vi "Git_UpdateApplicationPrep.vi"   [LabVIEW 2012]
uses:
  <vilib>/httpClient/LabVIEWHTTPClient.lvlib
  <vilib>/zip/NI_Unzip.lvlib
types:
  T1 = typedef "LabVIEWHTTPClient.lvlib/ClientHandle.ctl" = refnum<k1>
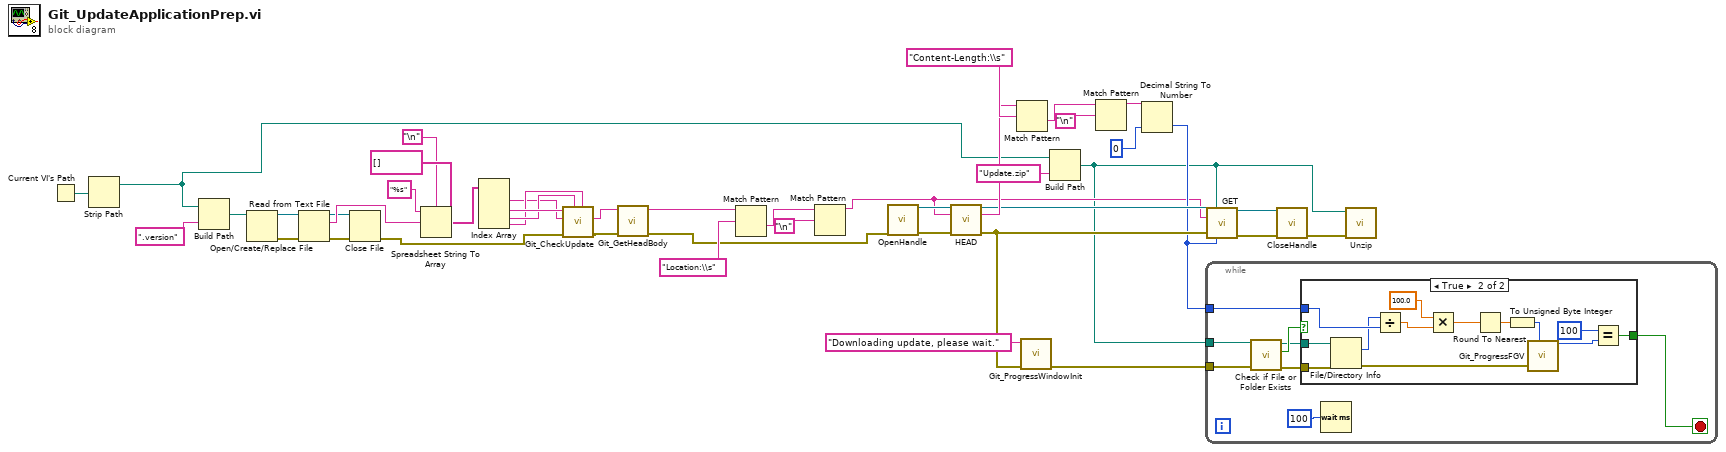
[diagram p0: block diagram]
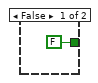
[diagram p2: hidden frame]
diagram:
  n1 = Current VI's Path() -> (path=w37:path)
  n2 = Strip Path(path=w37) -> (stripped path=w1:path)  [unwired: 1 out]
  n3 = Build Path(base path=w1, name or relative path=".version") -> (appended path=w43:path)
  n4 = Open/Create/Replace File(file path (use dialog)=w43) -> (refnum out=w41:refnum<file>, error out=w42:errorcluster)  [unwired: 5 in, 1 out]
  n5 = Read from Text File(file (use dialog)=w41, error in=w42) -> (refnum out=w29:refnum<file>, text=w39:string, error out=w31:errorcluster)  [unwired: 2 in, 1 out]
  n6 = Close File(refnum=w29, error in=w31) -> (error out=w30:errorcluster)  [unwired: 1 out]
  n7 = Spreadsheet String To Array(delimiter (Tab)="\n", format string="%s", spreadsheet string=w39, array type (2D Dbl)=string[] []) -> (array=w35:string[])
  n8 = Index Array(array=w35) -> (element #1=w28:string, element #2=w34:string, element #3=w33:string, element #4=w32:string)  [unwired: 4 in]
  n9 = call "Git_CheckUpdate.vi"("Current Version Date (YYYY-MM-DD)"=w32, "Current Version Number (vX.XX)"=w33, "error in"=w30, "Repo Name"=w28, "Repo User Name"=w34) -> ("error out"=w26:errorcluster, "Zip Address"=w27:string)  [unwired: 4 in, 1 out]
  n10 = call "Git_GetHeadBody.vi"("error in (no error)"=w26, "Address"=w27) -> ("error out"=w5:errorcluster, "headers"=w25:string)  [unwired: 7 in, 1 out]
  n11 = Match Pattern(string=w25, regular expression="Location:\\s") -> (after substring=w23:string)  [unwired: 1 in, 3 out]
  n12 = Match Pattern(string=w23, regular expression="\n") -> (before substring=w4:string)  [unwired: 1 in, 3 out]
  n13 = call <vilib>:"OpenHandle.vi"("error in (no error)"=w5) -> ("client handle out"=w21:T1, "error out"=w20:errorcluster)  [unwired: 13 in]
  n14 = call <vilib>:"HEAD.vi"("client handle"=w21, "url"=w4, "error in (no error)"=w20) -> ("client handle out"=w15:T1, "headers"=w16:string, "error out"=w13:errorcluster)  [unwired: 10 in]
  n15 = Match Pattern(string=w16, regular expression="Content-Length:\\s") -> (after substring=w18:string)  [unwired: 1 in, 3 out]
  n16 = call "Git_ProgressWindowInit.vi"("error in (no error)"=w13, "Message"="Downloading update, please wait.") -> ("error out"=w11:errorcluster)  [unwired: 7 in, 2 out]
  n17 = Build Path(base path=w1, name or relative path="Update.zip") -> (appended path=w2:path)
  n18 = Match Pattern(string=w18, regular expression="\n") -> (before substring=w10:string)  [unwired: 1 in, 3 out]
  n19 = Decimal String To Number(string=w10, default (0L)=i64 0) -> (number=w9:i64)  [unwired: 1 in, 1 out]
  n20 = while {
    tunnel: w11 -> [w49]
    tunnel: w2 -> [w45]
    tunnel: w9 -> [w51]
    stop <- w50 stop-if-true
    n21 = call <vilib>:"Check if File or Folder Exists.vi"("error in (no error)"=w49, "path"=w45) -> ("error out"=w48:errorcluster, "file or folder exists?"=w47:bool, "dup path"=w46:path)  [unwired: 7 in]
    n22 = case shown="True" w47 {
      tunnel: w51 -> [_ w64]
      tunnel: [FALSE w59] -> w50
      tunnel: w48 -> [_ w58]
      tunnel: w46 -> [_ w57]
      frame False {
      }
      frame True {
        n23 = File/Directory Info(path=w57, error in=w58) -> (size=w63:i64, error out=w65:errorcluster)  [unwired: 5 out]
        n24 = Divide(x=w63, y=w64) -> (x/y=w56:dbl)
        n25 = Multiply(x=100.0, y=w56) -> (x*y=w55:dbl)
        n26 = Round To Nearest(number=w55) -> (nearest integer value=w62:dbl)
        n27 = To Unsigned Byte Integer(number=w62) -> (unsigned 8bit integer=w61:u8)
        n28 = call "Git_ProgressFGV.vi"("Update"=w61, "Error In"=w65) -> ()  [unwired: 9 in, 1 out]
        n29 = Equal?(x=u8 100, y=w61) -> (x = y?=w59:bool)
      }
    }
    n30 = Wait (ms)(milliseconds to wait=u32 100) -> ()  [unwired: 1 out]
  }
  n31 = call <vilib>:"GET.vi"("client handle"=w15, "output file"=w2, "url"=w4, "error in (no error)"=w13, "timeout (10000)"=w9) -> ("client handle out"=w7:T1, "error out"=w8:errorcluster)  [unwired: 7 in, 2 out]
  n32 = call <vilib>:"CloseHandle.vi"("client handle"=w7, "error in (no error)"=w8) -> ("error out"=w3:errorcluster)  [unwired: 13 in]
  n33 = call <vilib>:"Unzip.vi"("error in (no error)"=w3, "Zip file"=w2) -> ()  [unwired: 7 in, 3 out]
